vi "Color_Sensor_Test.vi"() -> ()   [LabVIEW 2016]
panel:
  out "Robot Path":cluster{dbl[], dbl[]}[](graph)
  out "2D Picture":picture
  in  "Height":dbl
  in  "Y Location Sensor":dbl
  in  "X Location Sensor":dbl
  in  "Sensor Mode":u16(ring) items=["Ambient", "Detect", "Reflected"]
  out "Color Sensor Reading":dbl
  # "in"
  # "in"
  # "in"
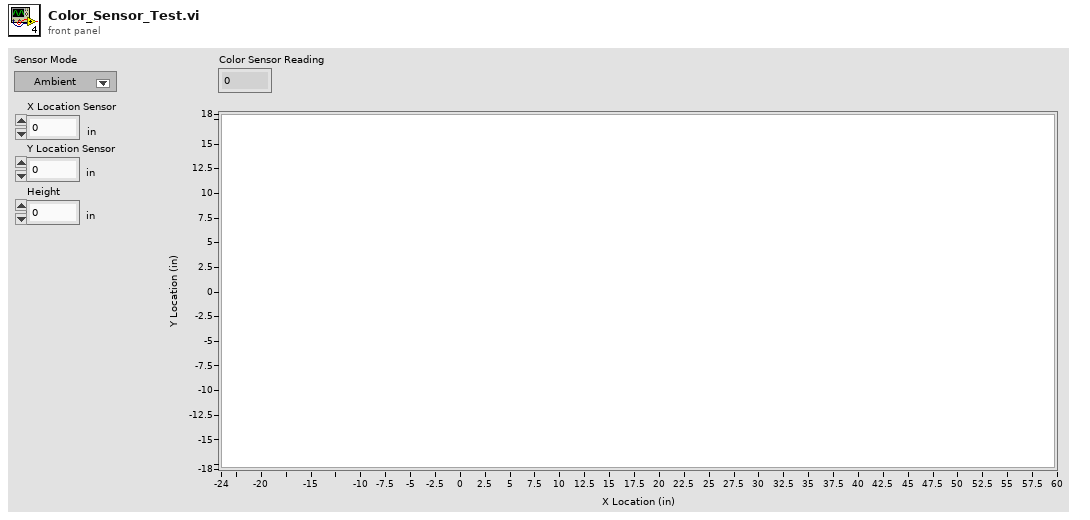
[diagram p1: front panel]
types:
  T1 = typedef "imagedata.ctl" = cluster{"image type":i32, "image depth":i32, "image":u8[], "mask":u8[], "colors":u32[], "Rectangle":cluster{"left":i16, "top":i16, "right":i16, "bottom":i16}}
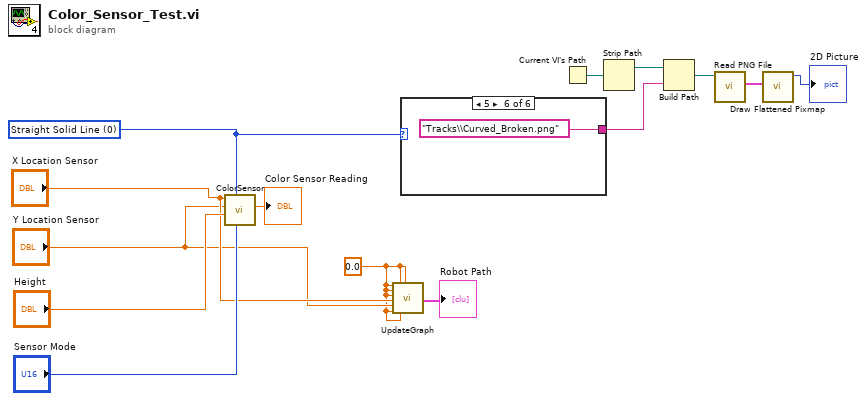
[diagram p0: block diagram]
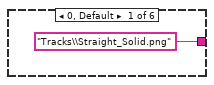
[diagram p2: hidden frame]
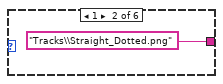
[diagram p3: hidden frame]
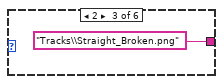
[diagram p4: hidden frame]
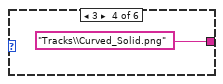
[diagram p5: hidden frame]
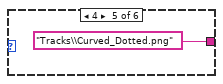
[diagram p6: hidden frame]
diagram:
  w1 = 0.0
  w6 = u16 0 items=["Straight Solid Line", "Straigh Dotted Line", "Straight Broken Line", "Curved Solid Line", "Curved Dotted Line", "Curved Broken Line"] ("Select Track")
  n1 = call "ColorSensor.vi"("Sensor Mode"="Sensor Mode", "Select Track"=w6, "Height"="Height", "Y Location Sensor"="Y Location Sensor", "X Location Sensor"="X Location Sensor") -> ("Color Sensor Reading"=→"Color Sensor Reading":dbl)  [unwired: 6 in]
  n2 = call "UpdateGraph.vi"("Angle"=w1, "Robot Length"=w1, "Robot Width"=w1, "Sensor 1 X"="X Location Sensor", "Sensor 1 Y"="Y Location Sensor", "Sensor 2 X"=w1, "Robot Y"=w1, "Sensor 2 Y"=w1, "Robot X"=w1) -> ("appended array"=→"Robot Path":cluster{dbl[], dbl[]}[])  [unwired: 10 in]
  n3 = case shown="5" w6 {
    tunnel: ["Tracks\\Straight_Solid.png" "Tracks\\Straight_Dotted.png" "Tracks\\Straight_Broken.png" "Tracks\\Curved_Solid.png" "Tracks\\Curved_Dotted.png" "Tracks\\Curved_Broken.png"] -> w10
    frame 0, Default {
    }
    frame 1 {
    }
    frame 2 {
    }
    frame 3 {
    }
    frame 4 {
    }
    frame 5 {
    }
  }
  n4 = Current VI's Path() -> (path=w11:path)
  n5 = Strip Path(path=w11) -> (stripped path=w7:path)  [unwired: 1 out]
  n6 = Build Path(base path=w7, name or relative path=w10) -> (appended path=w9:path)
  n7 = call <vilib>:"Read PNG File.vi"("path to PNG file"=w9) -> ("image data"=w8:T1)  [unwired: 8 in, 2 out]
  n8 = call <vilib>:"Draw Flattened Pixmap.vi"("image data"=w8) -> ("new picture"=→"2D Picture":picture)  [unwired: 8 in]
